vi "NIDAQGlobals.vi"() -> ()   [LabVIEW 2015]
panel:
  in  "Trigger Mode":enum16{"Normal", "One Red Frame Per Volume"}(ring)
  in  "Images per Volume":u16=1
  in  "Waveform Type":enum16{"Triangle", "Sawtooth"}(ring)
  in  "Volume Size":u16=1
  in  "Offset":dbl=-0.01
  in  "Dwell":u16=2
  in  "Frame Numbers":dbl[](array[numeric])
  out "DAQ Signals":dbl[][](array[numeric])=[[1.9650000000000158, 1.9650000000000158], [0.0, 0.0], [0.0, 0.0], [1.0, 1.0]]
  out "Scan Is Done":bool=TRUE
  out "Last Volume/Frame?":bool
  in  "Static Piezo Position":dbl=1.9650000000000158
  in  "Blue":dbl
  in  "Green":dbl=1.0
  in  "Red":dbl=1.0
  in  "DeltaZ":dbl=0.04
  in  "ZMin":dbl=2.5
  in  "ZMax":dbl=2.75
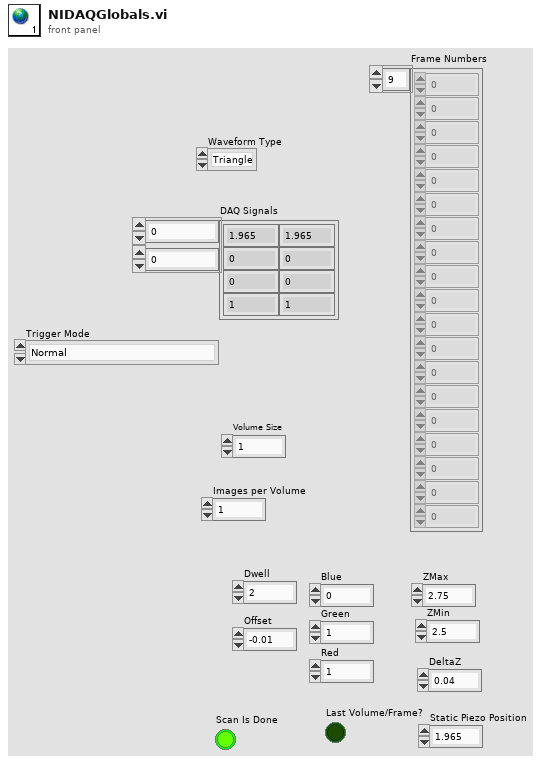
[diagram p1: front panel]
diagram:
